vi "Build Configuration Data.vi"(8 "error in (no error)":errorcluster, 11 "Configuration Window in":refnum<class "Configuration Window.lvclass">) -> (0 "error out":errorcluster, 2 "Configuration":T1={"Path Config"={"Data Folder Path"=path "", "PNG Folder Path"=path ""}, "Image Viewer Config"={"Center Point"={"Size"=3, "Color"=0, "Show?"=FALSE}, "bp Point"={"Size"=3, "Color"=0, "Show?"=FALSE}, "w Point"={"Size"=3, "Color"=0, "Show?"=FALSE}, "b Box"={"Fill Color"=0, "Border Color"=0, "Show?"=FALSE}, "i Box"={"Fill Color"=0, "Border Color"=0, "Show?"=FALSE}, "o Point"={"Size"=3, "Color"=0, "Show?"=FALSE}, "c Point"={"Size"=3, "Color"=0, "Show?"=FALSE}}}, 3 "Configuration Window out":refnum<class "Configuration Window.lvclass">)   [LabVIEW 2018, in "Configuration Window.lvlib" / "Configuration Window.lvclass"]
uses:
  Configuration Window.lvclass
  Main Panel/LF2R IDE/Const Configuration.ctl
  Main Panel/LF2R IDE/Const Path Setting.ctl
  Main Panel/LF2R IDE/Const Image Viewer Setting.ctl
  Configuration Window.lvclass/Configuration Window.ctl
  Main Panel/LF2R IDE/LF2R IDE.lvclass
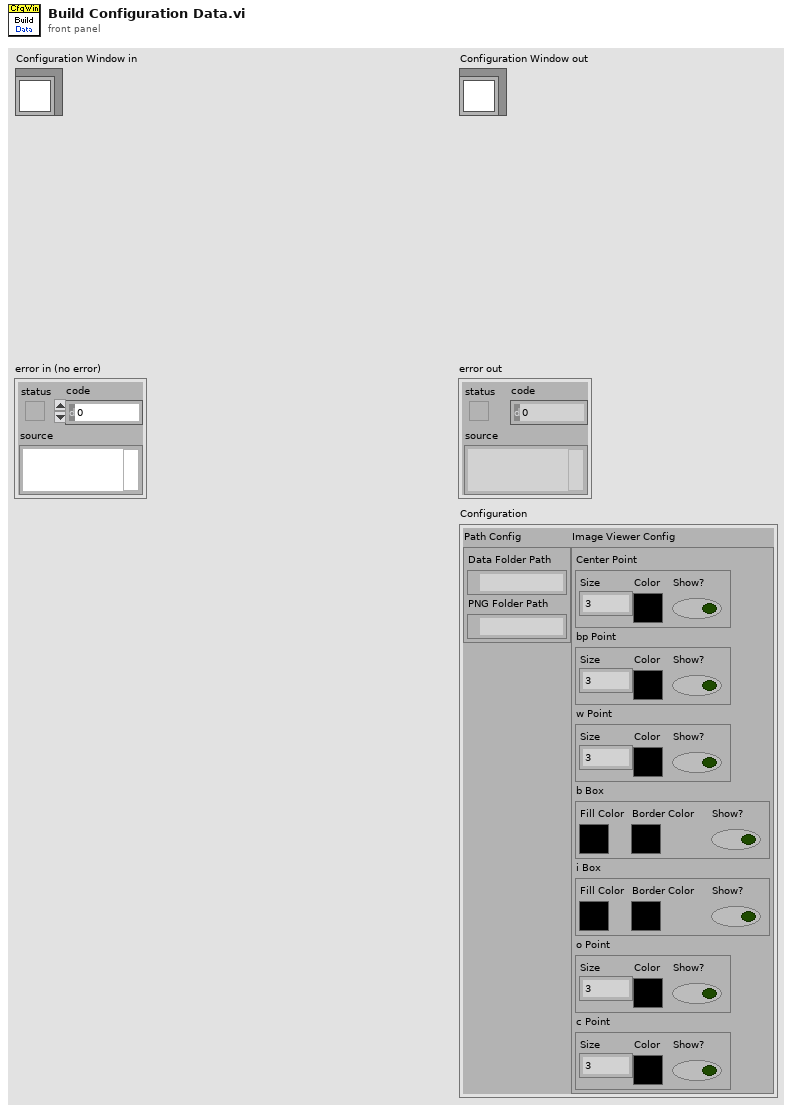
[diagram p1: front panel]
types:
  T1 = typedef "LF2R IDE.lvlib/LF2R IDE.lvclass/Const Configuration.ctl" = cluster{"Path Config":T2, "Image Viewer Config":T3}
  T2 = typedef "LF2R IDE.lvlib/LF2R IDE.lvclass/Const Path Setting.ctl" = cluster{"Data Folder Path":path, "PNG Folder Path":path}
  T3 = typedef "LF2R IDE.lvlib/LF2R IDE.lvclass/Const Image Viewer Setting.ctl" = cluster{"Center Point":cluster{"Size":i32, "Color":u32, "Show?":bool}, "bp Point":cluster{"Size":i32, "Color":u32, "Show?":bool}, "w Point":cluster{"Size":i32, "Color":u32, "Show?":bool}, "b Box":cluster{"Fill Color":u32, "Border Color":u32, "Show?":bool}, "i Box":cluster{"Fill Color":u32, "Border Color":u32, "Show?":bool}, "o Point":cluster{"Size":i32, "Color":u32, "Show?":bool}, "c Point":cluster{"Size":i32, "Color":u32, "Show?":bool}}
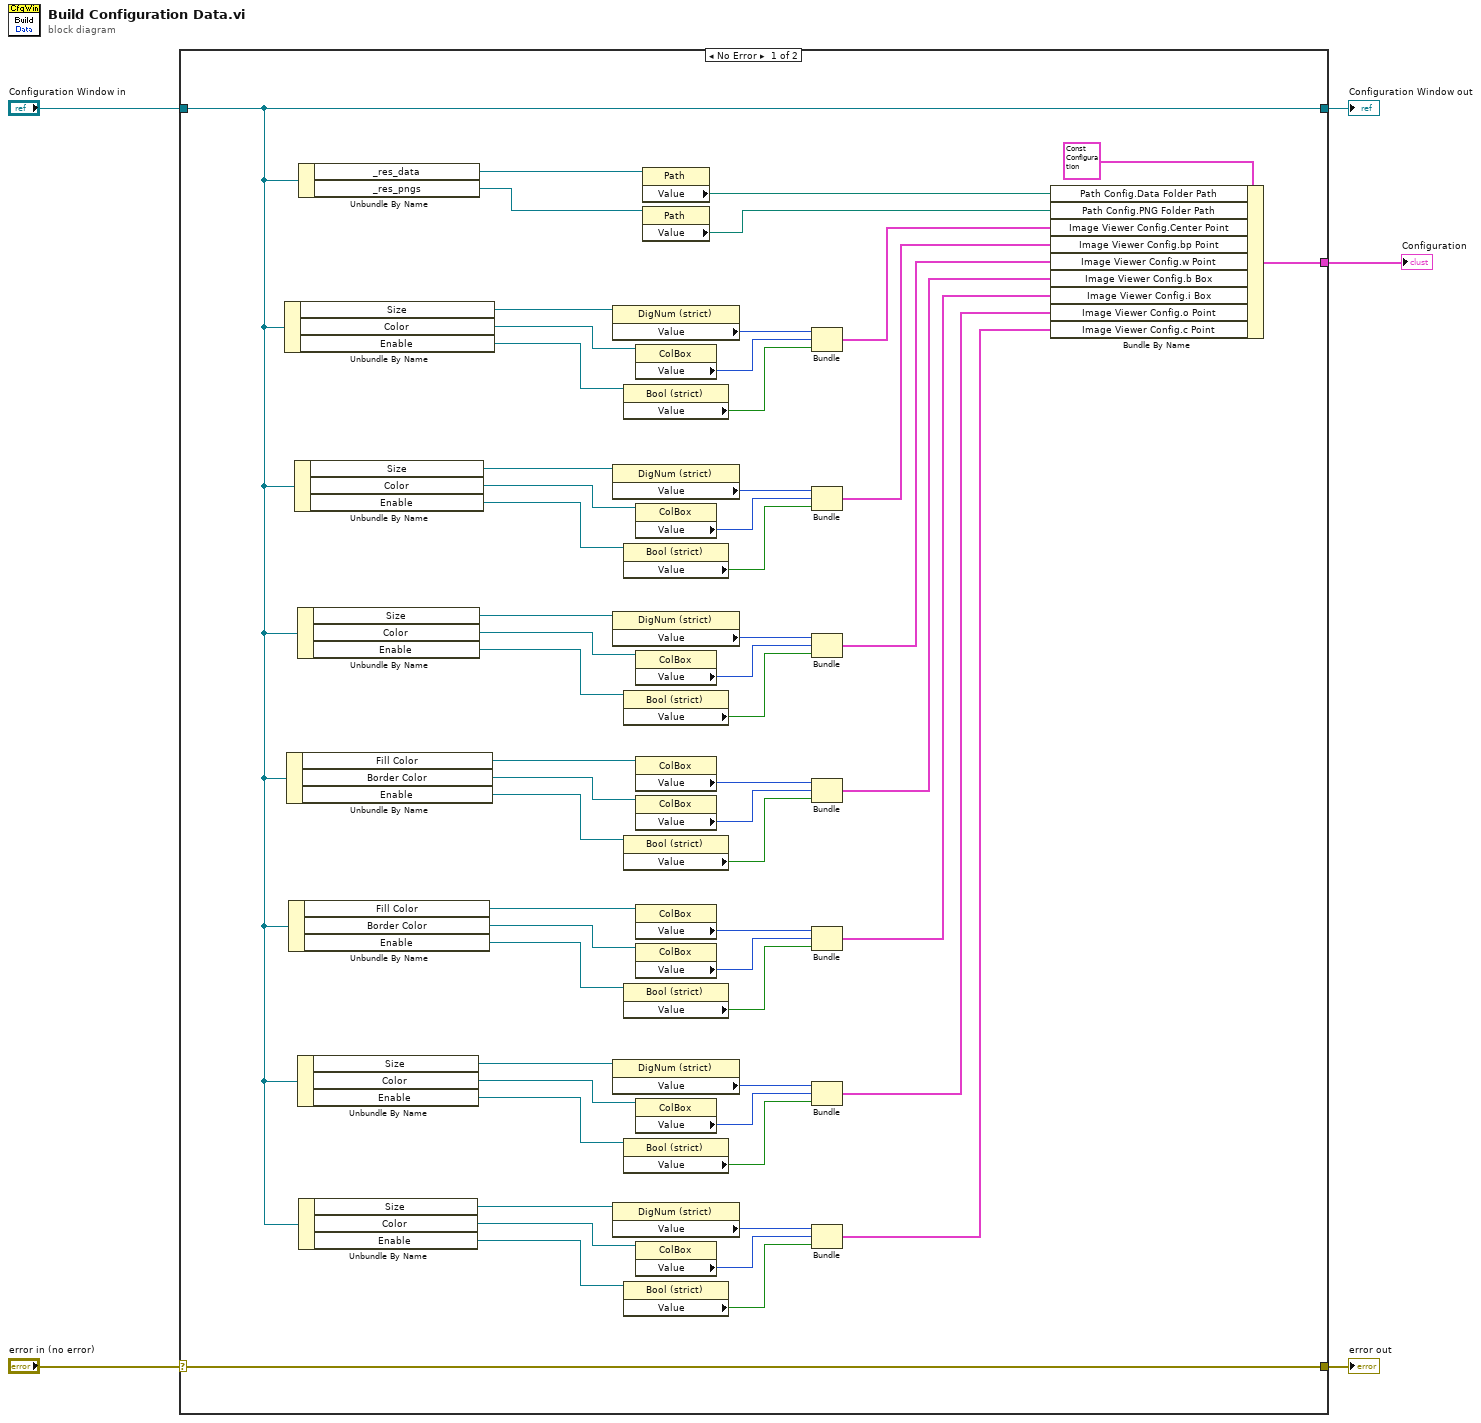
[diagram p0: block diagram]
diagram:
  n1 = case shown="No Error" "error in (no error)" {
    selector: "error in (no error)" -> [w62 w64]
    tunnel: [w62 w64] -> w4
    tunnel: [w10 w63] -> w2
    tunnel: "Configuration Window in" -> [w10 w63]
    tunnel: [w6 _] -> w1
    frame No Error {
      n2 = Unbundle By Name(w10) -> ("Size"=w56:refnum<vi>, "Color"=w55:refnum<vi>, "Enable"=w54:refnum<vi>)
      n3 = Unbundle By Name(w10) -> ("Fill Color"=w32:refnum<vi>, "Border Color"=w31:refnum<vi>, "Enable"=w30:refnum<vi>)
      n4 = Unbundle By Name(w10) -> ("Fill Color"=w28:refnum<vi>, "Border Color"=w24:refnum<vi>, "Enable"=w23:refnum<vi>)
      n5 = Unbundle By Name(w10) -> ("Size"=w44:refnum<vi>, "Color"=w45:refnum<vi>, "Enable"=w46:refnum<vi>)
      n6 = Unbundle By Name(w10) -> ("Size"=w42:refnum<vi>, "Color"=w38:refnum<vi>, "Enable"=w37:refnum<vi>)
      n7 = Unbundle By Name(w10) -> ("Size"=w18:refnum<vi>, "Color"=w17:refnum<vi>, "Enable"=w16:refnum<vi>)
      n8 = Unbundle By Name(w10) -> ("_res_data"=w61:refnum<vi>, "_res_pngs"=w58:refnum<vi>)
      n9 = Unbundle By Name(w10) -> ("Size"=w14:refnum<vi>, "Color"=w9:refnum<vi>, "Enable"=w8:refnum<vi>)
      n10 = property class="DigNum (strict)"(reference=w56) -> ("Value"=w53:i32)  [unwired: 1 in, 2 out]
      n11 = property class="DigNum (strict)"(reference=w44) -> ("Value"=w47:i32)  [unwired: 1 in, 2 out]
      n12 = property class="DigNum (strict)"(reference=w42) -> ("Value"=w41:i32)  [unwired: 1 in, 2 out]
      n13 = property class="DigNum (strict)"(reference=w18) -> ("Value"=w19:i32)  [unwired: 1 in, 2 out]
      n14 = property class="DigNum (strict)"(reference=w14) -> ("Value"=w13:i32)  [unwired: 1 in, 2 out]
      n15 = property class="Bool (strict)"(reference=w54) -> ("Value"=w51:bool)  [unwired: 1 in, 2 out]
      n16 = property class="Bool (strict)"(reference=w46) -> ("Value"=w49:bool)  [unwired: 1 in, 2 out]
      n17 = property class="Bool (strict)"(reference=w37) -> ("Value"=w39:bool)  [unwired: 1 in, 2 out]
      n18 = property class="Bool (strict)"(reference=w30) -> ("Value"=w35:bool)  [unwired: 1 in, 2 out]
      n19 = property class="Bool (strict)"(reference=w23) -> ("Value"=w25:bool)  [unwired: 1 in, 2 out]
      n20 = property class="Bool (strict)"(reference=w16) -> ("Value"=w21:bool)  [unwired: 1 in, 2 out]
      n21 = property class="Bool (strict)"(reference=w8) -> ("Value"=w11:bool)  [unwired: 1 in, 2 out]
      n22 = property class="ColBox"(reference=w55) -> ("Value"=w52:u32)  [unwired: 1 in, 2 out]
      n23 = property class="ColBox"(reference=w45) -> ("Value"=w48:u32)  [unwired: 1 in, 2 out]
      n24 = property class="ColBox"(reference=w38) -> ("Value"=w40:u32)  [unwired: 1 in, 2 out]
      n25 = property class="ColBox"(reference=w32) -> ("Value"=w33:u32)  [unwired: 1 in, 2 out]
      n26 = property class="ColBox"(reference=w31) -> ("Value"=w34:u32)  [unwired: 1 in, 2 out]
      n27 = property class="ColBox"(reference=w28) -> ("Value"=w27:u32)  [unwired: 1 in, 2 out]
      n28 = property class="ColBox"(reference=w24) -> ("Value"=w26:u32)  [unwired: 1 in, 2 out]
      n29 = property class="ColBox"(reference=w17) -> ("Value"=w20:u32)  [unwired: 1 in, 2 out]
      n30 = property class="ColBox"(reference=w9) -> ("Value"=w12:u32)  [unwired: 1 in, 2 out]
      n31 = property class="Path"(reference=w61) -> ("Value"=w59:path)  [unwired: 1 in, 2 out]
      n32 = property class="Path"(reference=w58) -> ("Value"=w57:path)  [unwired: 1 in, 2 out]
      n33 = Bundle("Value"=w53, "Value"=w52, "Value"=w51) -> (w50:cluster{"Value":i32, "Value":u32, "Value":bool})  [unwired: 1 in]
      n34 = Bundle("Value"=w47, "Value"=w48, "Value"=w49) -> (w43:cluster{"Value":i32, "Value":u32, "Value":bool})  [unwired: 1 in]
      n35 = Bundle("Value"=w41, "Value"=w40, "Value"=w39) -> (w36:cluster{"Value":i32, "Value":u32, "Value":bool})  [unwired: 1 in]
      n36 = Bundle("Value"=w33, "Value"=w34, "Value"=w35) -> (w29:cluster{"Value":u32, "Value":u32, "Value":bool})  [unwired: 1 in]
      n37 = Bundle("Value"=w27, "Value"=w26, "Value"=w25) -> (w22:cluster{"Value":u32, "Value":u32, "Value":bool})  [unwired: 1 in]
      n38 = Bundle("Value"=w19, "Value"=w20, "Value"=w21) -> (w15:cluster{"Value":i32, "Value":u32, "Value":bool})  [unwired: 1 in]
      n39 = Bundle("Value"=w13, "Value"=w12, "Value"=w11) -> (w7:cluster{"Value":i32, "Value":u32, "Value":bool})  [unwired: 1 in]
      n40 = Bundle By Name(cluster=T1 {"Path Config"={"Data Folder Path"=path "", "PNG Folder Path"=path ""}, "Image Viewer Config"={"Center Point"={"Size"=3, "Color"=0, "Show?"=FALSE}, "bp Point"={"Size"=3, "Color"=0, "Show?"=FALSE}, "w Point"={"Size"=3, "Color"=0, "Show?"=FALSE}, "b Box"={"Fill Color"=0, "Border Color"=0, "Show?"=FALSE}, "i Box"={"Fill Color"=0, "Border Color"=0, "Show?"=FALSE}, "o Point"={"Size"=3, "Color"=0, "Show?"=FALSE}, "c Point"={"Size"=3, "Color"=0, "Show?"=FALSE}}} ("Configuration 2"), "Path Config.Data Folder Path"=w59, "Path Config.PNG Folder Path"=w57, "Image Viewer Config.Center Point"=w50, "Image Viewer Config.bp Point"=w43, "Image Viewer Config.w Point"=w36, "Image Viewer Config.b Box"=w29, "Image Viewer Config.i Box"=w22, "Image Viewer Config.o Point"=w15, "Image Viewer Config.c Point"=w7) -> (w6:T1)
    }
    frame Error {
    }
  }
  "error out" <- w4
  "Configuration Window out" <- w2
  "Configuration" <- w1
